vi "FGV_PSP - IPS120 Mode Status.vi"(4 "error in":errorcluster, 6 "Function":enum16{"write", "read"}(ring), 7 "Mode":T1) -> (0 "error out":errorcluster, 3 "Mode":T1)   [LabVIEW 2016, in "IPS-120.lvlib" / "IPS-120-API.lvlib"]
uses:
  IPS-120-API.lvlib
  IPS120/Typedefs/Read Mode 2 - Enum.ctl
  IPS-120.lvlib
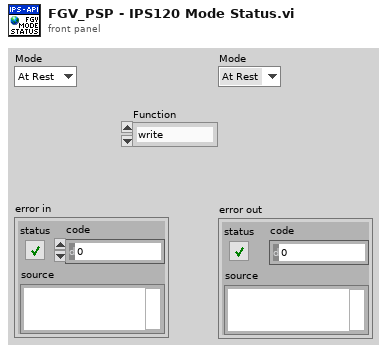
[diagram p1: front panel]
types:
  T1 = typedef "IPS-120.lvlib/Read Mode 2 - Enum.ctl" = enum16{"At Rest", "Sweeping", "Sweep Limiting", "Sweeping & Sweep Limiting"}
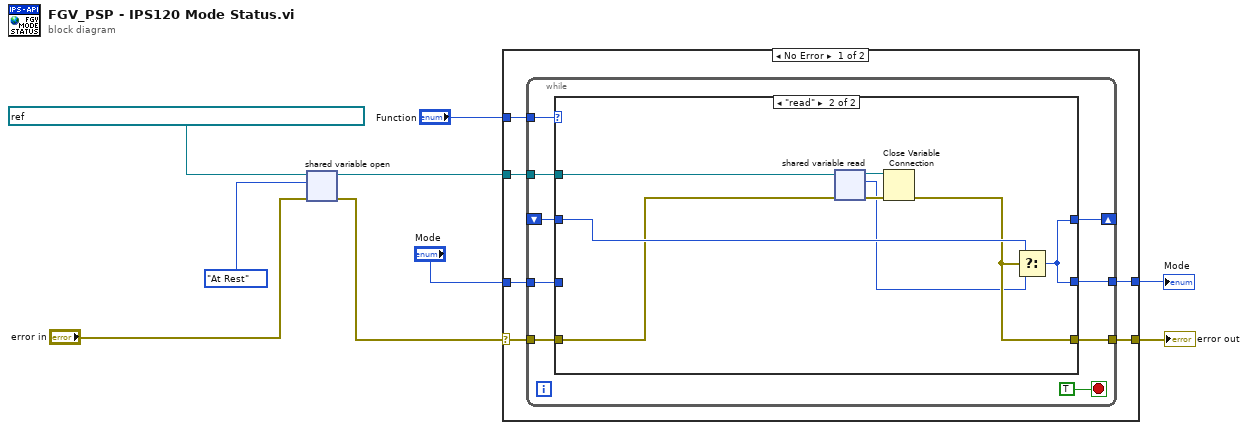
[diagram p0: block diagram]
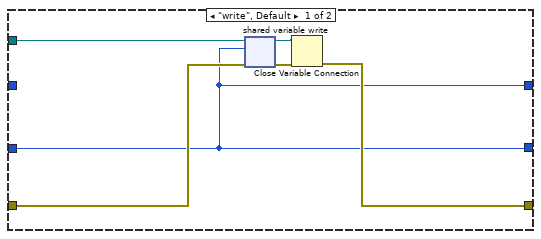
[diagram p2: hidden frame]
diagram:
  n1 = shared-variable-open(refnum<k21> "ni.var.psp://localhost/IPS120/ModeStatus" ("shared variable refnum in"), "error in", Read_Mode_2_-_Enum."At Rest" ("Mode 2")) -> (w7:refnum<k21>, w5:errorcluster)  [unwired: 1 in]
  n2 = case shown="No Error" w5 {
    selector: w5 -> [w15 w40]
    tunnel: [w14 w40] -> w9
    tunnel: [w13 w39] -> w2
    tunnel: "Function" -> [w12 _]
    tunnel: w7 -> [w11 _]
    tunnel: "Mode" -> [w10 w39]
    frame No Error {
      n3 = while {
        shift-right: [w19] -> _
        shift-left: _ -> [w18]
        tunnel: w15 -> [w23]
        tunnel: [w22] -> w14
        tunnel: [w21] -> w13
        tunnel: w12 -> [w20]
        tunnel: w11 -> [w17]
        tunnel: w10 -> [w16]
        stop <- TRUE stop-if-true
        n4 = case shown="\"read\"" w20 {
          tunnel: w23 -> [w27 w32]
          tunnel: [w29 w34] -> w22
          tunnel: [w25 w35] -> w21
          tunnel: [w25 w35] -> w19
          tunnel: w18 -> [_ w36]
          tunnel: w17 -> [w26 w33]
          tunnel: w16 -> [w25 _]
          frame "write", Default {
            n5 = shared-variable-write(w26, w27, w25) -> (w28:refnum<k21>, w30:errorcluster)
            n6 = Close Variable Connection(8:w30, 11:w28) -> (0:w29:errorcluster)
          }
          frame "read" {
            n7 = shared-variable-read(w33, w32) -> (w38:refnum<k21>, w37:errorcluster, w31:T1)  [unwired: 1 out]
            n8 = Close Variable Connection(8:w37, 11:w38) -> (0:w34:errorcluster)
            n9 = Select(t=w36, s=w34, f=w31) -> (s? t:f=w35:T1)
          }
        }
      }
    }
    frame Error {
    }
  }
  "error out" <- w9
  "Mode" <- w2
